vi "Untitled 16.vi"() -> ()   [LabVIEW 2013]
uses:
  JSONtext.lvlib
panel:
  out "data":cluster{"Polynomial Coefficients":dbl[]}
  out "error out":errorcluster
  out "Variant out":variant
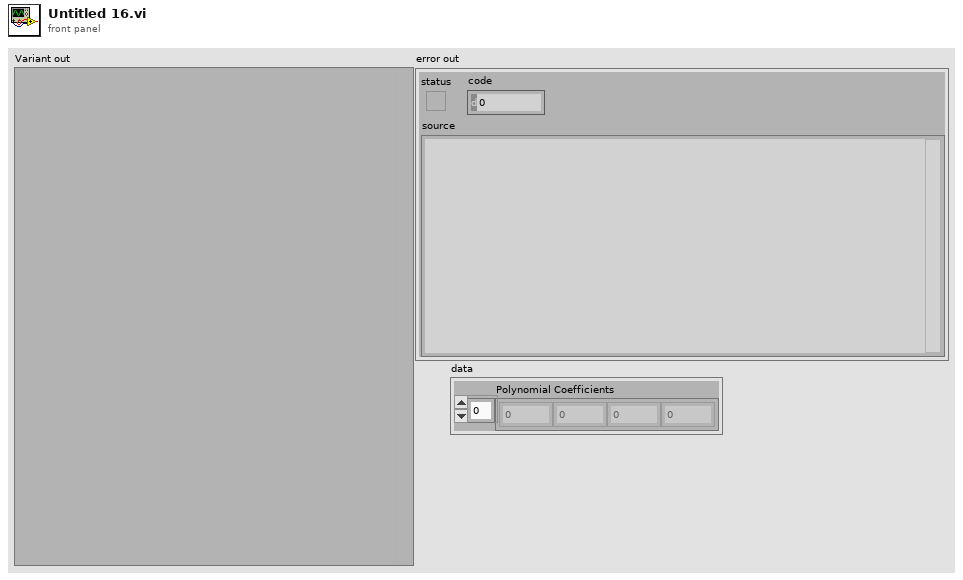
[diagram p1: front panel]
types:
  T1 = cluster{"Other Variables":cluster{"Name":string, "Value":dbl}[]}
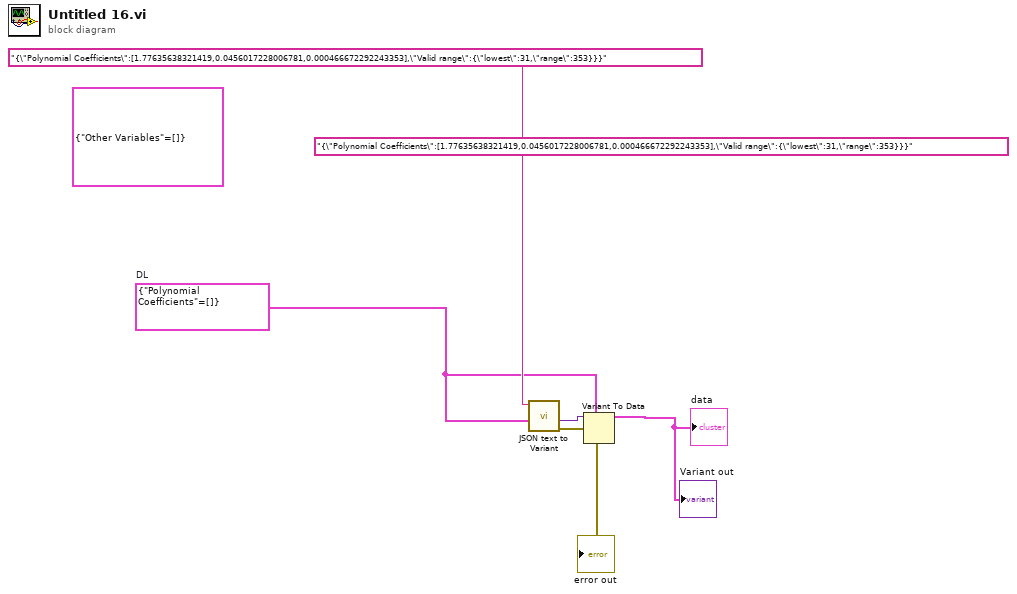
[diagram p0: block diagram]
diagram:
  (unwired) "{\"Polynomial Coefficients\":[1.77635638321419,0.0456017228006781,0.000466672292243353],\"Valid range\":{\"lowest\":31,\"range\":353}}}"
  w2 = cluster{"Polynomial Coefficients":dbl[]} {"Polynomial Coefficients"=[]}  # DL
  (unwired) T1 {"Other Variables"=[]}
  n1 = call "JSON text to Variant.vi"("Variant (Data Type)"=w2, "JSON"="{\"Polynomial Coefficients\":[1.77635638321419,0.0456017228006781,0.000466672292243353],\"Valid range\":{\"lowest\":31,\"range\":353}}}") -> ("error out"=→"error out":errorcluster, "Variant out"=w4:variant)  [unwired: 8 in]
  n2 = Variant To Data(type=w2, Variant=w4) -> (data=→"Variant out" →"data":cluster{"Polynomial Coefficients":dbl[]})  [unwired: 1 in, 1 out]
